vi "GlobalMiscellaneous.vi"() -> ()   [LabVIEW 2020]
doc: "This global variable contains current robot state information and actuator setpoints."
panel:
  out "Swerve_Output_Loop_Time (ms)":u32
  out "REF_LEDs":string
  out "CON_Robot_Code_Version":string
  out "Pose_Loop_Time (ms)":u32
  out "Control_Latency_Alarm":bool
  out "Control_Loop_Time (ms)":u32
  out "SEN_CAN_Bus_Fault":bool
  out "SEN_Battery_Critical":bool
  out "SEN_Electrical_Fault":bool
  out "SEN_Battery_Voltage (V)":dbl
  out "SEN_Pressure_Vent":bool
  out "SEN_Pressure_Leak":bool
  out "SEN_Compressor_On":bool
  out "SEN_Pressure_Transducer (PSI)":dbl
  out "CON_Robot_Profile":string
  out "CON_PDH_Current_Channels":cluster{string, dbl}[](array[cluster])=[{"", 0.0}, {"Climber Motor Left", 0.0}, {"Module 3 Azimuth", 0.0}, {"Module 3 Drive", 0.0}, {"Module 2 Azimuth", 0.0}, {"Module 2 Drive", 0.0}, {"Tower Motor", 0.0}, {"Turret Motor", 0.0}, {"Kicker Motor", 0.0}, {"Pneumatics Hub", 0.0}, {"Cowl Motor", 0.0}, {"Shooter Motor Lower", 0.0}, {"Shooter Motor Upper", 0.0}, {"Module 1 Azimuth", 0.0}, {"Module 1 Drive", 0.0}, {"Intake Motor Right", 0.0}, {"Indexer Motor", 0.0}, {"Intake Motor Left", 0.0}, {"Module 0 Drive", 0.0}, {"Module 0 Azimuth", 0.0}, {"Radio Power Module", 0.0}, {"RobotRIO", 0.0}, {"LimeLight", 0.0}, {"LED Spotlights", 0.0}]
  out "CON_Legal_Actuator_Names":string[](array[string])
  out "CON_Number_of_LEDs":u16
  out "REF_Compressor":string
  out "Master_Caution":bool
  out "Number_of_Master_Alarms":i32
  out "Master_Alarm":bool
  out "LimeLight_PiP_Mode":T1(ring)
  out "Diverting_Power_LimeLight":bool
  out "LimeLight_Pipeline_Commanded":T2(ring)
  out "LED_Colors":u32[](array[colorbox])
  out "LimeLight_LED_Mode":enum16{"Pipeline Setting", "Off", "Blink", "On"}(ring)=enum."Off"
  out "Diverting_Power_LEDS":bool
  out "Disallowed_Master_States":bool[](array[boolean])
  out "Diverting_Power_Compressor":bool
  out "Confirmed_Master_States":bool[](array[boolean])
  # "MASTER STATE CONTROLLER"
  # "PRESSURE MANAGEMENT"
  # "COMPUTE RESOURCES"
  # "ALARM MANAGEMENT"
  # "DEVICE REFERENCES"
  # "CONSTANTS"
  # "OUTPUTS"
  # "POWER MANAGEMENT"
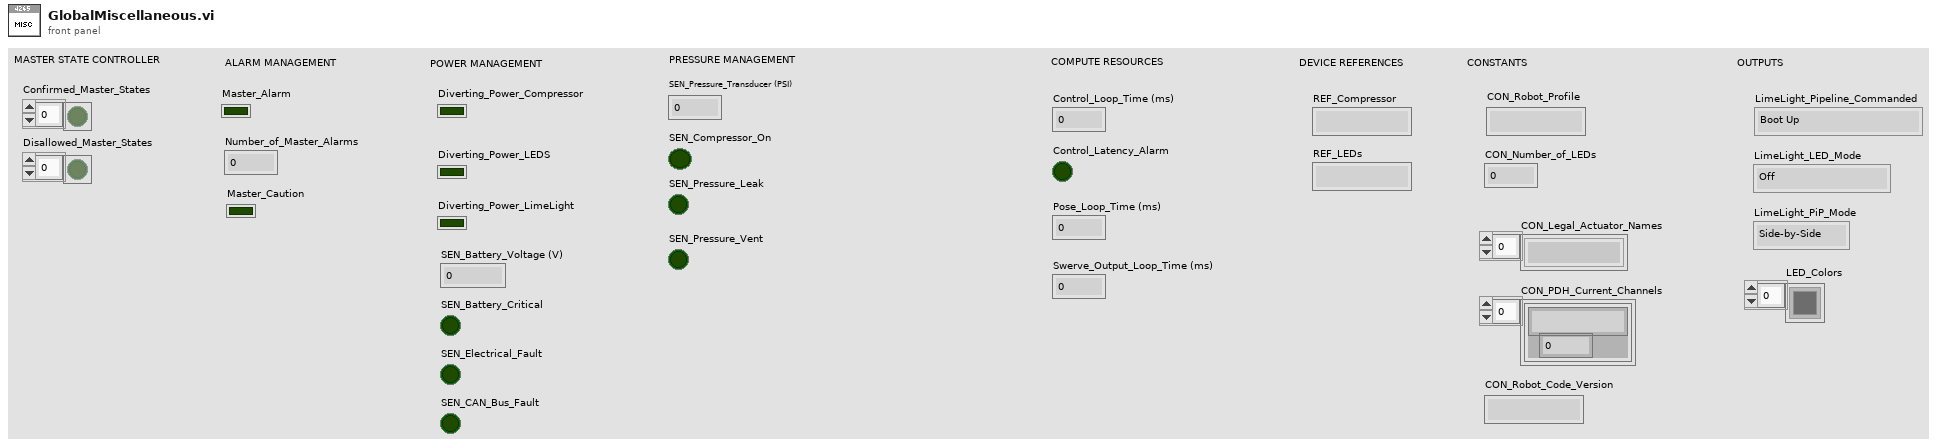
[diagram p1: front panel]
types:
  T1 = enum16{"Side-by-Side", "PiP Main", "PiP Secondary"}
  T2 = enum16{"Boot Up", "Camera Override", "AprilTags", "Gamepiece Tracking"}
diagram:
